vi "svx_Autoscale Ranges.vi"(7 "Plot Area:Size:Width":u32, 10 "Display State In":T4={"X Scale Width %"=50.0, "Y Scale Height %"=50.0, "X-Axis Range"={"Minimum"=0.0, "Maximum"=10.0}, "Y-Axis Range"={"Minimum"=0.0, "Maximum"=10.0}, "Z-Axis Range"={"Minimum"=0.0, "Maximum"=10.0}, "Plot Color"=61212, "Frame Color"=16252785, "Background Color"=16777222, "Initial AutoScale Y"=TRUE, "AutoScale X"=2, "AutoScale Y"=2, "AutoScale Z"=2, "Plot Transparency"=FALSE, "X-Axis Name"="Frequency", "Y-Axis Name"="Amplitude", "Z-Axis Name"="", "X-Axis Scaling Factor"={"Offset"=0.0, "Multiplier"=1.0}, "Y-Axis Scaling Factor"={"Offset"=0.0, "Multiplier"=1.0}, "Z-Axis Scaling Factor"={"Offset"=0.0, "Multiplier"=1.0}, "X-Scale Visible"=TRUE, "Y-Scale Visible"=TRUE, "Z-Scale Visible"=TRUE, "X-Scale Label Visible"=TRUE, "Y-Scale Label Visible"=TRUE, "Z-Scale Label Visible"=TRUE, "X-Axis Range Scaled"={"Minimum"=0.0, "Maximum"=10.0}, "Y-Axis Range Scaled"={"Minimum"=0.0, "Maximum"=10.0}, "Z-Axis Range Scaled"={"Minimum"=0.0, "Maximum"=10.0}, "Rev Z Order"=FALSE, "X-Scale Format Str"="%#.4g", "Y-Scale Format Str"="%#.4g", "Z-Scale Format Str"="%#.4g", "Decor color"=12369084, "Scale Range Change"=refnum, "out of state queue"=refnum, "property nodes"=refnum, "Lines"=[], "Line Properties"={"Line Color"=61212, "Line Width"=61212, "Line Style"=enum."Dash", "DisplayLines"=FALSE}} {"Line Properties"."Line Width" min=1}, 11 "Data Array In":T2={"z0"=0.0, "dz"=1.0, "Plots"=[]}) -> (0 "Cropped Info out":cluster{"First Index":i32, "Length":i32}, 1 "Update Ranges":bool[](array[boolean]), 2 "Display State Out":T4={"X Scale Width %"=50.0, "Y Scale Height %"=50.0, "X-Axis Range"={"Minimum"=0.0, "Maximum"=10.0}, "Y-Axis Range"={"Minimum"=0.0, "Maximum"=10.0}, "Z-Axis Range"={"Minimum"=0.0, "Maximum"=10.0}, "Plot Color"=61212, "Frame Color"=16252785, "Background Color"=16777222, "Initial AutoScale Y"=TRUE, "AutoScale X"=2, "AutoScale Y"=2, "AutoScale Z"=2, "Plot Transparency"=FALSE, "X-Axis Name"="Frequency", "Y-Axis Name"="Amplitude", "Z-Axis Name"="", "X-Axis Scaling Factor"={"Offset"=0.0, "Multiplier"=1.0}, "Y-Axis Scaling Factor"={"Offset"=0.0, "Multiplier"=1.0}, "Z-Axis Scaling Factor"={"Offset"=0.0, "Multiplier"=1.0}, "X-Scale Visible"=TRUE, "Y-Scale Visible"=TRUE, "Z-Scale Visible"=TRUE, "X-Scale Label Visible"=TRUE, "Y-Scale Label Visible"=TRUE, "Z-Scale Label Visible"=TRUE, "X-Axis Range Scaled"={"Minimum"=0.0, "Maximum"=10.0}, "Y-Axis Range Scaled"={"Minimum"=0.0, "Maximum"=10.0}, "Z-Axis Range Scaled"={"Minimum"=0.0, "Maximum"=10.0}, "Rev Z Order"=FALSE, "X-Scale Format Str"="%#.4g", "Y-Scale Format Str"="%#.4g", "Z-Scale Format Str"="%#.4g", "Decor color"=12369084, "Scale Range Change"=refnum, "out of state queue"=refnum, "property nodes"=refnum, "Lines"=[], "Line Properties"={"Line Color"=61212, "Line Width"=61212, "Line Style"=enum."Dash", "DisplayLines"=FALSE}} {"Line Properties"."Line Width" min=1}, 3 "Dec/Cropped and Lines Out":T1={"Dec/Cropped in"={"z0"=0.0, "dz"=1.0, "Plots"=[]}, "Lines"=[]}, 4 "Update Autoscale":bool)   [LabVIEW 2017, in "SVX Waterfall Graph.xctl"]
uses:
  <vilib>/addons/_XControls/Waterfall Graph/SVX Waterfall Graph.xctl
  <vilib>/addons/_XControls/Waterfall Graph/subVIs/svx_Waterfall Data.ctl
  <vilib>/addons/_XControls/Waterfall Graph/subVIs/svx_CroppedData.ctl
  <vilib>/addons/_NISVFA/_Shared subVIs/Controls/svc_Cluster of Array of Cluster of XYZ.ctl
  <vilib>/addons/_XControls/Waterfall Graph/subVIs/svx_Waterfall State.ctl
panel:
  in  "Dec/Cropped and Lines In":T1={"Dec/Cropped in"={"z0"=0.0, "dz"=1.0, "Plots"=[]}, "Lines"=[]}
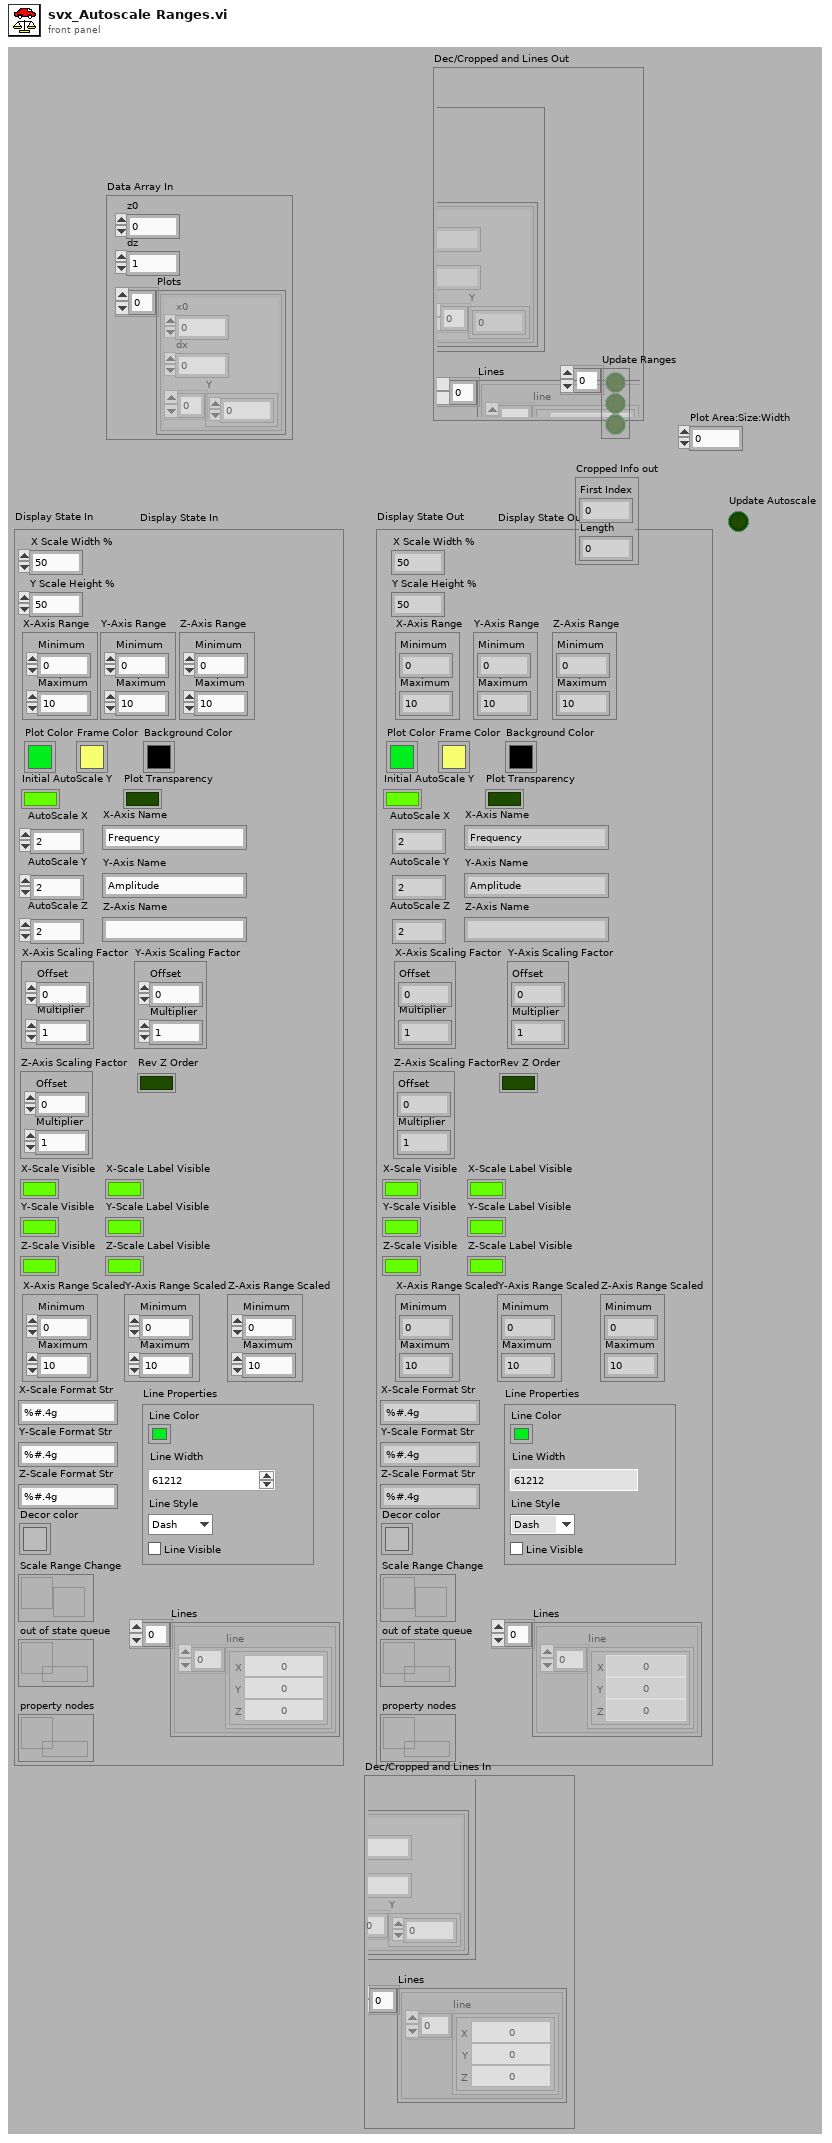
[diagram p1: front panel]
types:
  T1 = typedef "SVX Waterfall Graph.xctl/svx_CroppedData.ctl" = cluster{"Dec/Cropped in":T2, "Lines":T3[]}
  T2 = typedef "SVX Waterfall Graph.xctl/svx_Waterfall Data.ctl" = cluster{"z0":dbl, "dz":dbl, "Plots":cluster{"x0":dbl, "dx":dbl, "Y":dbl[]}[]}
  T3 = typedef "svc_Cluster of Array of Cluster of XYZ.ctl" = cluster{"line":cluster{"X":dbl, "Y":dbl, "Z":dbl}[]}
  T4 = typedef "SVX Waterfall Graph.xctl/svx_Waterfall State.ctl" = cluster{"X Scale Width %":dbl, "Y Scale Height %":dbl, "X-Axis Range":cluster{"Minimum":dbl, "Maximum":dbl}, "Y-Axis Range":cluster{"Minimum":dbl, "Maximum":dbl}, "Z-Axis Range":cluster{"Minimum":dbl, "Maximum":dbl}, "Plot Color":u32, "Frame Color":u32, "Background Color":u32, "Initial AutoScale Y":bool, "AutoScale X":u8, "AutoScale Y":u8, "AutoScale Z":u8, "Plot Transparency":bool, "X-Axis Name":string, "Y-Axis Name":string, "Z-Axis Name":string, "X-Axis Scaling Factor":cluster{"Offset":dbl, "Multiplier":dbl}, "Y-Axis Scaling Factor":cluster{"Offset":dbl, "Multiplier":dbl}, "Z-Axis Scaling Factor":cluster{"Offset":dbl, "Multiplier":dbl}, "X-Scale Visible":bool, "Y-Scale Visible":bool, "Z-Scale Visible":bool, "X-Scale Label Visible":bool, "Y-Scale Label Visible":bool, "Z-Scale Label Visible":bool, "X-Axis Range Scaled":cluster{"Minimum":dbl, "Maximum":dbl}, "Y-Axis Range Scaled":cluster{"Minimum":dbl, "Maximum":dbl}, "Z-Axis Range Scaled":cluster{"Minimum":dbl, "Maximum":dbl}, "Rev Z Order":bool, "X-Scale Format Str":string, "Y-Scale Format Str":string, "Z-Scale Format Str":string, "Decor color":u32, "Scale Range Change":refnum<user-event>, "out of state queue":refnum<queue>, "property nodes":refnum<queue>, "Lines":T3[], "Line Properties":cluster{"Line Color":u32, "Line Width":u16, "Line Style":enum32{"Solid", "Dash", "Dot", "DashDot", "DashDotDot"}, "DisplayLines":bool}}
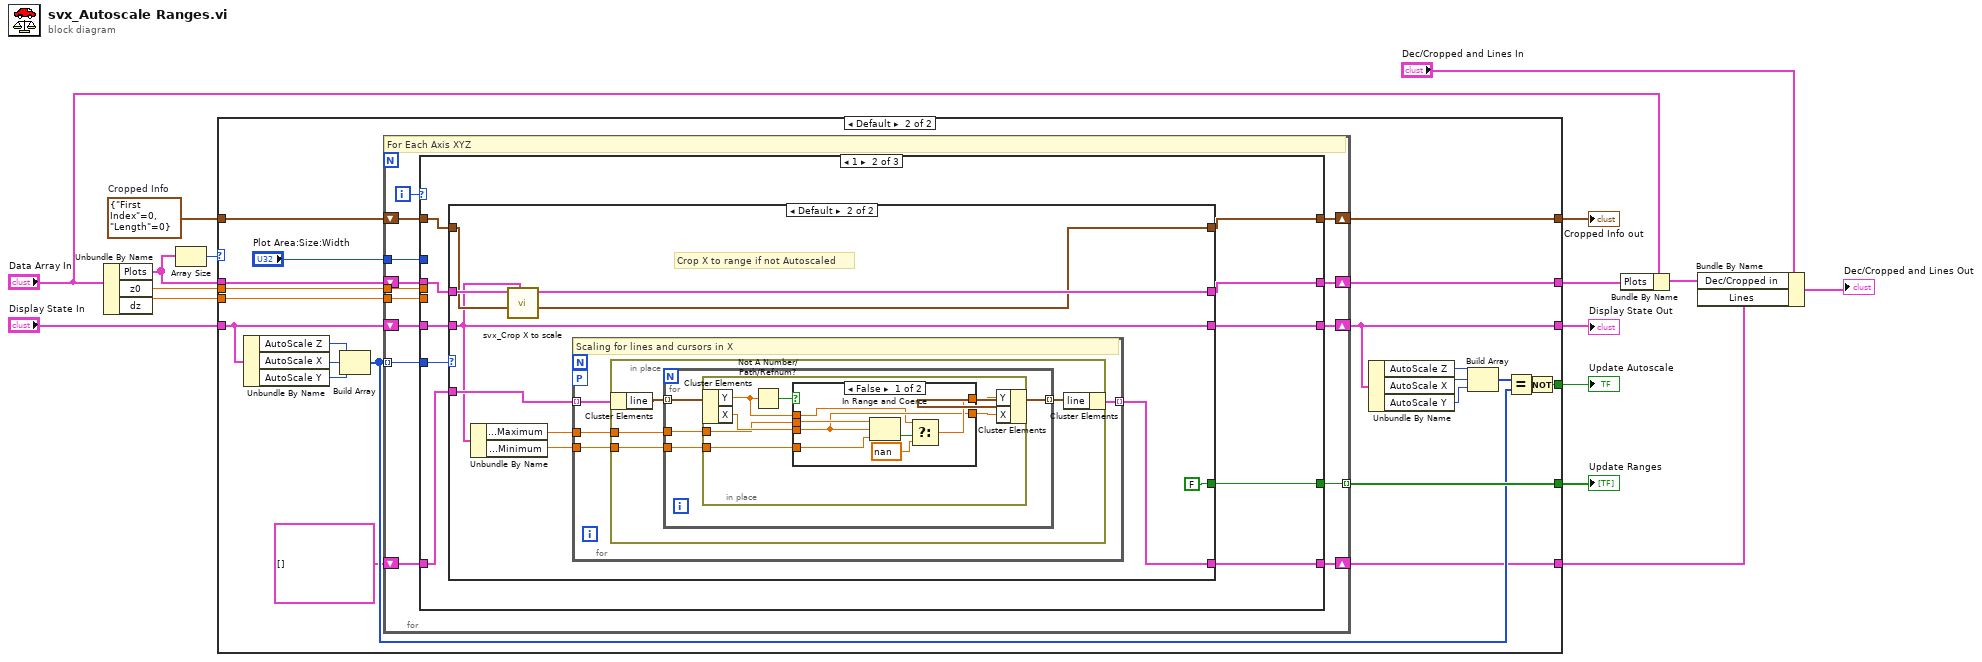
[diagram p0: block diagram]
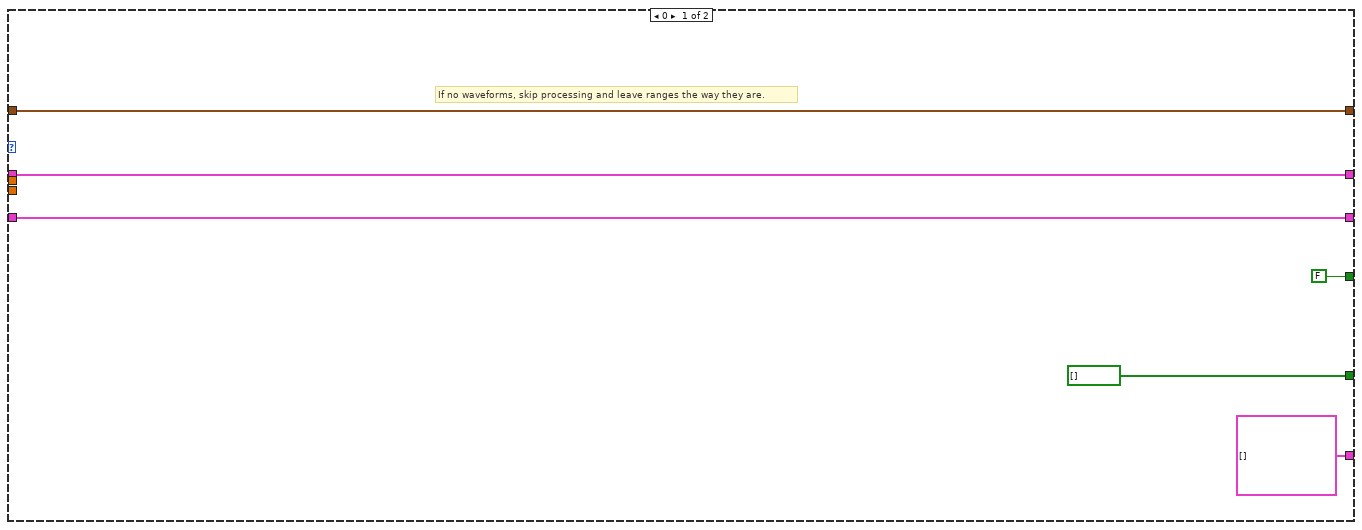
[diagram p2: hidden frame]
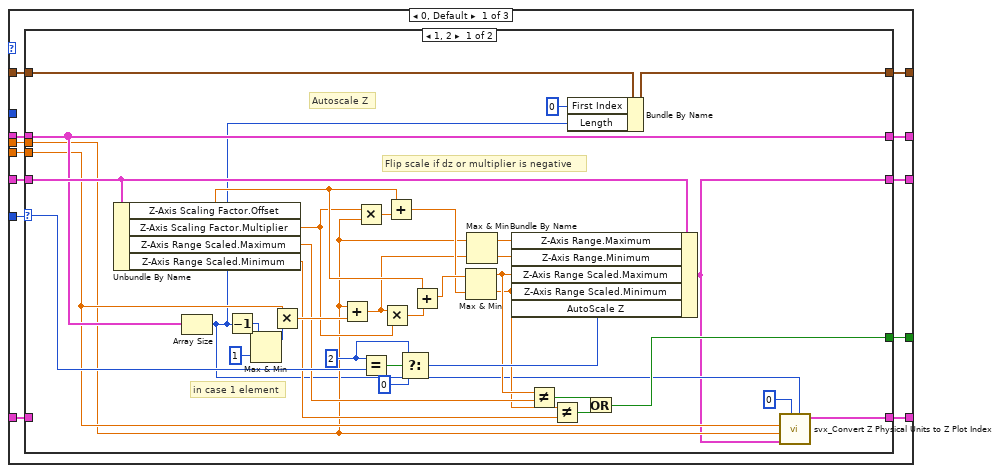
[diagram p3: hidden frame]
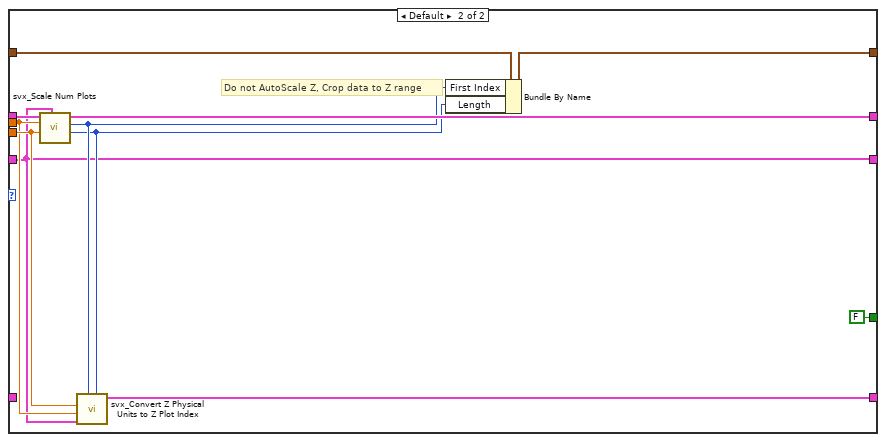
[diagram p4: hidden frame]
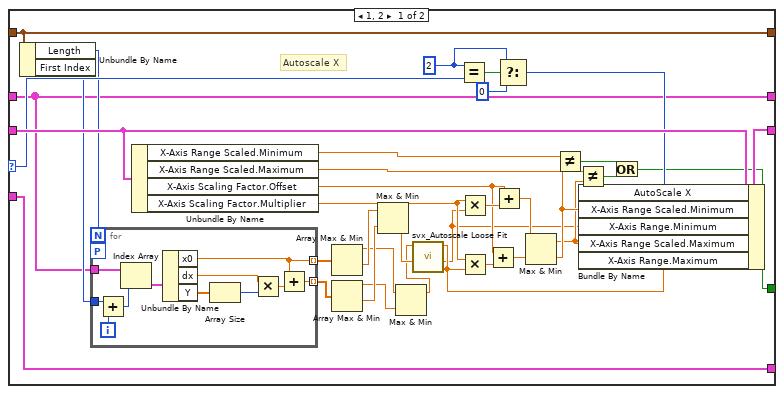
[diagram p5: hidden frame]
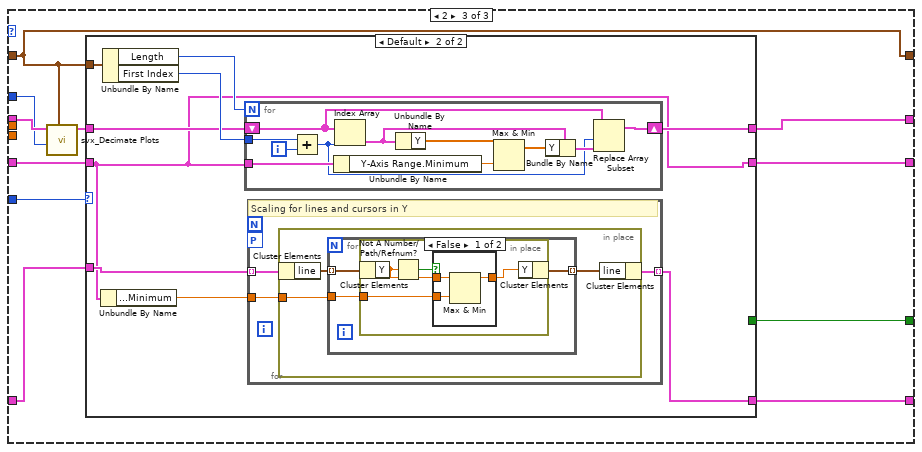
[diagram p7: hidden frame]
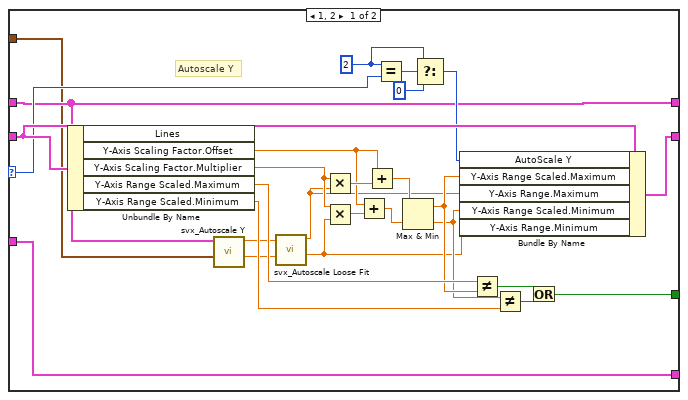
[diagram p8: hidden frame]
diagram:
  w12 = cluster{"First Index":i32, "Length":i32} {"First Index"=0, "Length"=0}  # Cropped Info
  n1 = Unbundle By Name("Data Array In") -> ("Plots"=w11:cluster{"x0":dbl, "dx":dbl, "Y":dbl[]}[], "z0"=w8:dbl, "dz"=w7:dbl)
  n2 = Array Size(array=w11) -> (size(s)=w15:i32)
  n3 = case shown="Default" w15 {
    tunnel: [w21 w30] -> w2
    tunnel: "Display State In" -> [w21 w44]
    tunnel: w11 -> [w22 w40]
    tunnel: [w22 w39] -> w9
    tunnel: [bool[] [] w38] -> w14
    tunnel: [w19 w37] -> w13
    tunnel: w12 -> [w19 w36]
    tunnel: w8 -> [_ w25]
    tunnel: w7 -> [_ w26]
    tunnel: [FALSE w27] -> w6
    tunnel: [T3[] [] ("Lines") w23] -> w1
    frame 0 {
      # "If no waveforms, skip processing and leave ranges the way they are."
    }
    frame Default {
      n4 = Unbundle By Name(w44) -> ("AutoScale Z"=w43:u8, "AutoScale X"=w42:u8, "AutoScale Y"=w41:u8)
      n5 = Build Array(w43, w42, w41) -> (w29:u8[])
      n6 = for {
        shift-right: [w47] -> w30
        shift-left: w44 -> [w58]
        tunnel: w29 -> [w55] mode=indexing
        shift-right: [w54] -> w39
        shift-left: w40 -> [w57]
        tunnel: [w53] -> w38 mode=indexing
        shift-right: [w51] -> w37
        shift-left: w36 -> [w52]
        tunnel: w25 -> [w50]
        tunnel: w26 -> [w48]
        tunnel: "Plot Area:Size:Width" -> [w49]
        shift-right: [w46] -> w23
        shift-left: T3[] [] ("Lines") -> [w45]
        i -> [w56]
        # "For Each Axis XYZ"
        n7 = case shown="1" w56 {
          tunnel: w58 -> [w70 w127 w222]
          tunnel: [w69 w120 w221] -> w47
          tunnel: w57 -> [w68 w126 w217]
          tunnel: w55 -> [w67 w125 w220]
          tunnel: [w66 w124 w219] -> w54
          tunnel: [w65 w123 w218] -> w53
          tunnel: w52 -> [w64 w122 w215]
          tunnel: [w63 w121 w215] -> w51
          tunnel: w50 -> [w62 _ _]
          tunnel: w48 -> [w61 _ _]
          tunnel: w49 -> [_ _ w214]
          tunnel: [w60 w118 w212] -> w46
          tunnel: w45 -> [w59 w119 w213]
          frame 0, Default {
            n8 = case shown="1, 2" w67 {
              selector: w67 -> [w92 _]
              tunnel: w70 -> [w106 w107]
              tunnel: [w71 w107] -> w69
              tunnel: w68 -> [w80 w117]
              tunnel: [w80 w116] -> w66
              tunnel: [w84 FALSE] -> w65
              tunnel: w64 -> [w83 w114]
              tunnel: [w82 w113] -> w63
              tunnel: w62 -> [w75 w111]
              tunnel: w61 -> [w76 w112]
              tunnel: [w72 w108] -> w60
              tunnel: w59 -> [_ _]
              frame 1, 2 {
                w94 = u8 2 ("AutoScale Y")
                # "in case 1 element"
                # "Flip scale if dz or multiplier is negative"
                # "Autoscale Z"
                n9 = Unbundle By Name(w106) -> ("Z-Axis Scaling Factor.Offset"=w103:dbl, "Z-Axis Scaling Factor.Multiplier"=w101:dbl, "Z-Axis Range Scaled.Maximum"=w88:dbl, "Z-Axis Range Scaled.Minimum"=w86:dbl)
                n10 = Array Size(array=w80) -> (size(s)=w73:i32)
                n11 = Decrement(x=w73) -> (x-1=w79:i32)
                n12 = Max & Min(x=w79, y=1) -> (max(x,y)=w78:i32)  [unwired: 1 out]
                n13 = Multiply(x=w76, y=w78) -> (x*y=w102:dbl)
                n14 = Add(x=w75, y=w102) -> (x+y=w98:dbl)
                n15 = Multiply(x=w101, y=w75) -> (x*y=w105:dbl)
                n16 = Equal?(x=w94, y=w92) -> (x = y?=w95:bool)
                n17 = Multiply(x=w98, y=w101) -> (x*y=w104:dbl)
                n18 = Add(x=w103, y=w105) -> (x+y=w99:dbl)
                n19 = Select(t=w94, s=w95, f=u8 0 ("AutoScale Y")) -> (s? t:f=w91:u8)
                n20 = Add(x=w103, y=w104) -> (x+y=w100:dbl)
                n21 = Max & Min(x=w100, y=w99) -> (max(x,y)=w87:dbl, min(x,y)=w85:dbl)
                n22 = Max & Min(x=w75, y=w98) -> (max(x,y)=w97:dbl, min(x,y)=w96:dbl)
                n23 = Bundle By Name(cluster=w106, "Z-Axis Range.Maximum"=w97, "Z-Axis Range.Minimum"=w96, "Z-Axis Range Scaled.Maximum"=w87, "Z-Axis Range Scaled.Minimum"=w85, "AutoScale Z"=w91) -> (w71:T4)
                n24 = Not Equal?(x=w87, y=w88) -> (x != y?=w90:bool)
                n25 = Not Equal?(x=w85, y=w86) -> (x != y?=w89:bool)
                n26 = Bundle By Name(cluster=w83, "First Index"=0, "Length"=w73) -> (w82:cluster{"First Index":i32, "Length":i32})
                n27 = Or(x=w90, y=w89) -> (x .or. y?=w84:bool)
                n28 = call <vilib>:"svx_Convert Z Physical Units to Z Plot Index.vi"("Z length"=w73, "Z Index"=0 ("First Index"), "Display State In"=w71, "z0"=w75, "dz"=w76) -> ("Lines"=w72:T3[])  [unwired: 6 in]
              }
              frame Default {
                # "Do not AutoScale Z, Crop data to Z range"
                n29 = call <vilib>:"svx_Scale Num Plots.vi"("Display State In"=w107, "dz"=w112, "z0"=w111, "Plots"=w117) -> ("Z length"=w109:i32, "Z Index"=w110:i32, "Plots out"=w116:cluster{"x0":dbl, "dx":dbl, "Y":dbl[]}[])  [unwired: 5 in]
                n30 = call <vilib>:"svx_Convert Z Physical Units to Z Plot Index.vi"("Z length"=w109, "Z Index"=w110, "Display State In"=w107, "z0"=w111, "dz"=w112) -> ("Lines"=w108:T3[])  [unwired: 6 in]
                n31 = Bundle By Name(cluster=w114, "First Index"=w110, "Length"=w109) -> (w113:cluster{"First Index":i32, "Length":i32})
              }
            }
          }
          frame 1 {
            n32 = case shown="Default" w125 {
              selector: w125 -> [w145 _]
              tunnel: w127 -> [w161 w174]
              tunnel: [w162 w174] -> w120
              tunnel: w126 -> [w129 w180]
              tunnel: [w129 w183] -> w124
              tunnel: [w138 FALSE ("Boolean")] -> w123
              tunnel: w122 -> [w136 w177]
              tunnel: [w136 w181] -> w121
              tunnel: w119 -> [w128 w176]
              tunnel: [w128 w175] -> w118
              frame 1, 2 {
                w147 = u8 2 ("AutoScale Y")
                # "Autoscale X"
                n33 = Unbundle By Name(w136) -> ("Length"=w135:i32, "First Index"=w134:i32)
                n34 = for {
                  N: w135 -> [_]
                  tunnel: [w169] -> w154 mode=indexing
                  tunnel: [w168] -> w153 mode=indexing
                  tunnel: w129 -> [w167]
                  tunnel: w134 -> [w164]
                  workers-P: _ -> [_]
                  i -> [w165]
                  n35 = Add(x=w164, y=w165) -> (x+y=w163:i32)
                  n36 = Index Array(array=w167, index=w163) -> (element=w166:cluster{"x0":dbl, "dx":dbl, "Y":dbl[]})
                  n37 = Unbundle By Name(w166) -> ("x0"=w169:dbl, "dx"=w171:dbl, "Y"=w173:dbl[])
                  n38 = Array Size(array=w173) -> (size(s)=w172:i32)
                  n39 = Multiply(x=w171, y=w172) -> (x*y=w170:dbl)
                  n40 = Add(x=w169, y=w170) -> (x+y=w168:dbl)
                }
                n41 = Unbundle By Name(w161) -> ("X-Axis Range Scaled.Minimum"=w137:dbl, "X-Axis Range Scaled.Maximum"=w142:dbl, "X-Axis Scaling Factor.Offset"=w157:dbl, "X-Axis Scaling Factor.Multiplier"=w158:dbl)
                n42 = Array Max & Min(array=w154) -> (max value=w150:dbl, min value=w152:dbl)  [unwired: 2 out]
                n43 = Array Max & Min(array=w153) -> (max value=w149:dbl, min value=w151:dbl)  [unwired: 2 out]
                n44 = Max & Min(x=w152, y=w151) -> (min(x,y)=w133:dbl)  [unwired: 1 out]
                n45 = Max & Min(x=w150, y=w149) -> (max(x,y)=w132:dbl)  [unwired: 1 out]
                n46 = call <vilib>:"svx_Autoscale Loose Fit.vi"("Min"=w133, "Max"=w132) -> ("Loose Fit Min"=w130:dbl, "Loose Fit Max"=w131:dbl)  [unwired: 8 in]
                n47 = Equal?(x=w147, y=w145) -> (x = y?=w148:bool)
                n48 = Multiply(x=w158, y=w130) -> (x*y=w160:dbl)
                n49 = Multiply(x=w158, y=w131) -> (x*y=w159:dbl)
                n50 = Add(x=w157, y=w159) -> (x+y=w156:dbl)
                n51 = Add(x=w157, y=w160) -> (x+y=w155:dbl)
                n52 = Select(t=w147, s=w148, f=u8 0 ("AutoScale Y")) -> (s? t:f=w144:u8)
                n53 = Max & Min(x=w155, y=w156) -> (max(x,y)=w141:dbl, min(x,y)=w143:dbl)
                n54 = Not Equal?(x=w137, y=w143) -> (x != y?=w140:bool)
                n55 = Not Equal?(x=w142, y=w141) -> (x != y?=w139:bool)
                n56 = Bundle By Name(cluster=w161, "AutoScale X"=w144, "X-Axis Range Scaled.Minimum"=w143, "X-Axis Range.Minimum"=w130, "X-Axis Range Scaled.Maximum"=w141, "X-Axis Range.Maximum"=w131) -> (w162:T4)
                n57 = Or(x=w140, y=w139) -> (x .or. y?=w138:bool)
              }
              frame Default {
                # "Crop X to range if not Autoscaled"
                n58 = Unbundle By Name(w174) -> ("X-Axis Range.Maximum"=w179:dbl, "X-Axis Range.Minimum"=w178:dbl)
                n59 = call <vilib>:"svx_Crop X to scale.vi"("Display State In"=w174, "Cropped Info"=w177, "Plots"=w180) -> ("Cropped Info out"=w181:cluster{"First Index":i32, "Length":i32}, "Plots"=w183:cluster{"x0":dbl, "dx":dbl, "Y":dbl[]}[])  [unwired: 7 in]
                n60 = for {
                  tunnel: w176 -> [w186] mode=indexing
                  tunnel: w179 -> [w187]
                  tunnel: [w185] -> w175 mode=indexing
                  tunnel: w178 -> [w184]
                  workers-P: _ -> [_]
                  # "Scaling for lines and cursors in X"
                  n61 = in-place {
                    in-place-border: w187 -> [w191]
                    in-place-border: w184 -> [w188]
                    n62 = in-place-cluster #1(w186) -> ("line"=w190:cluster{"X":dbl, "Y":dbl, "Z":dbl}[])
                    n63 = for {
                      tunnel: w190 -> [w195] mode=indexing
                      tunnel: w191 -> [w194]
                      tunnel: [w193] -> w189 mode=indexing
                      tunnel: w188 -> [w192]
                      n64 = in-place {
                        in-place-border: w194 -> [w198]
                        in-place-border: w192 -> [w197]
                        n65 = in-place-cluster #2(w195) -> ("Y"=w201:dbl, "X"=w199:dbl)
                        n66 = Not A Number/Path/Refnum?(number/path/refnum=w201) -> (NaN/Path/Refnum?=w202:bool)
                        n67 = case shown="False" w202 {
                          tunnel: w201 -> [w203 w211]
                          tunnel: [w208 w211] -> w200
                          tunnel: w199 -> [w204 w210]
                          tunnel: w198 -> [w206 _]
                          tunnel: w197 -> [w207 _]
                          tunnel: [w204 w210] -> w196
                          frame False {
                            n68 = In Range and Coerce(upper limit=w206, x=w204, lower limit=w207) -> (In Range?=w209:bool)  [unwired: 1 out]
                            n69 = Select(t=w203, s=w209, f=nan) -> (s? t:f=w208:dbl)
                          }
                          frame True {
                            # "Y is NaN"
                          }
                        }
                        n70 = in-place-cluster #2("Y"=w200, "X"=w196) -> (w193:cluster{"X":dbl, "Y":dbl, "Z":dbl})
                      }
                    }
                    n71 = in-place-cluster #1("line"=w189) -> (w185:T3)
                  }
                }
              }
            }
          }
          frame 2 {
            n72 = call <vilib>:"svx_Decimate Plots.vi"("Cropped Info"=w215, "Width"=w214, "Plots"=w217) -> ("Plots out"=w216:cluster{"x0":dbl, "dx":dbl, "Y":dbl[]}[])  [unwired: 8 in]
            n73 = case shown="Default" w220 {
              selector: w220 -> [w241 _]
              tunnel: w222 -> [w248 w251]
              tunnel: [w249 w251] -> w221
              tunnel: w216 -> [w227 w254]
              tunnel: [w227 w255] -> w219
              tunnel: [w230 FALSE] -> w218
              tunnel: w215 -> [w226 w258]
              tunnel: w213 -> [w223 w252]
              tunnel: [w223 w250] -> w212
              frame 1, 2 {
                w239 = u8 2 ("AutoScale Y")
                # "Autoscale Y"
                n74 = Unbundle By Name(w248) -> ("Y-Axis Scaling Factor.Offset"=w244:dbl, "Y-Axis Scaling Factor.Multiplier"=w245:dbl, "Y-Axis Range Scaled.Maximum"=w234:dbl, "Y-Axis Range Scaled.Minimum"=w232:dbl)  [unwired: 1 out]
                n75 = call <vilib>:"svx_Autoscale Y.vi"("Cropped Info"=w226, "Plots"=w227) -> ("min"=w224:dbl, "max"=w225:dbl)  [unwired: 8 in]
                n76 = call <vilib>:"svx_Autoscale Loose Fit.vi"("Min"=w224, "Max"=w225) -> ("Loose Fit Min"=w228:dbl, "Loose Fit Max"=w229:dbl)  [unwired: 8 in]
                n77 = Multiply(x=w245, y=w229) -> (x*y=w247:dbl)
                n78 = Multiply(x=w245, y=w228) -> (x*y=w246:dbl)
                n79 = Add(x=w244, y=w246) -> (x+y=w243:dbl)
                n80 = Add(x=w244, y=w247) -> (x+y=w242:dbl)
                n81 = Equal?(x=w239, y=w241) -> (x = y?=w240:bool)
                n82 = Max & Min(x=w242, y=w243) -> (max(x,y)=w233:dbl, min(x,y)=w231:dbl)
                n83 = Select(t=w239, s=w240, f=u8 0 ("AutoScale Y")) -> (s? t:f=w237:u8)
                n84 = Bundle By Name(cluster=w248, "AutoScale Y"=w237, "Y-Axis Range Scaled.Maximum"=w233, "Y-Axis Range.Maximum"=w229, "Y-Axis Range Scaled.Minimum"=w231, "Y-Axis Range.Minimum"=w228) -> (w249:T4)
                n85 = Not Equal?(x=w234, y=w233) -> (x != y?=w236:bool)
                n86 = Not Equal?(x=w231, y=w232) -> (x != y?=w235:bool)
                n87 = Or(x=w236, y=w235) -> (x .or. y?=w230:bool)
              }
              frame Default {
                n88 = Unbundle By Name(w251) -> ("Y-Axis Range.Minimum"=w253:dbl)
                n89 = Unbundle By Name(w258) -> ("Length"=w257:i32, "First Index"=w256:i32)
                n90 = for {
                  N: w257 -> [_]
                  tunnel: w251 -> [w287]
                  tunnel: w256 -> [w281]
                  shift-right: [w279] -> w255
                  shift-left: w254 -> [w278]
                  i -> [w282]
                  n91 = Add(x=w281, y=w282) -> (x+y=w277:i32)
                  n92 = Unbundle By Name(w287) -> ("Y-Axis Range.Minimum"=w285:dbl)
                  n93 = Index Array(array=w278, index=w277) -> (element=w283:cluster{"x0":dbl, "dx":dbl, "Y":dbl[]})
                  n94 = Unbundle By Name(w283) -> ("Y"=w286:dbl[])
                  n95 = Max & Min(x=w286, y=w285) -> (max(x,y)=w284:dbl[])  [unwired: 1 out]
                  n96 = Bundle By Name(cluster=w283, "Y"=w284) -> (w280:cluster{"x0":dbl, "dx":dbl, "Y":dbl[]})
                  n97 = Replace Array Subset(array=w278, new element=w280, index=w277) -> (w279:cluster{"x0":dbl, "dx":dbl, "Y":dbl[]}[])
                }
                n98 = for {
                  tunnel: w252 -> [w261] mode=indexing
                  tunnel: w253 -> [w262]
                  tunnel: [w260] -> w250 mode=indexing
                  workers-P: _ -> [_]
                  # "Scaling for lines and cursors in Y"
                  n99 = in-place {
                    in-place-border: w262 -> [w265]
                    n100 = in-place-cluster #3(w261) -> ("line"=w264:cluster{"X":dbl, "Y":dbl, "Z":dbl}[])
                    n101 = for {
                      tunnel: w264 -> [w268] mode=indexing
                      tunnel: w265 -> [w267]
                      tunnel: [w266] -> w263 mode=indexing
                      n102 = in-place {
                        in-place-border: w267 -> [w269]
                        n103 = in-place-cluster #4(w268) -> ("Y"=w271:dbl)
                        n104 = Not A Number/Path/Refnum?(number/path/refnum=w271) -> (NaN/Path/Refnum?=w272:bool)
                        n105 = case shown="False" w272 {
                          tunnel: w271 -> [w275 w276]
                          tunnel: [w273 w276] -> w270
                          tunnel: w269 -> [w274 _]
                          frame False {
                            n106 = Max & Min(x=w275, y=w274) -> (max(x,y)=w273:dbl)  [unwired: 1 out]
                          }
                          frame True {
                            # "NaN"
                          }
                        }
                        n107 = in-place-cluster #4("Y"=w270) -> (w266:cluster{"X":dbl, "Y":dbl, "Z":dbl})
                      }
                    }
                    n108 = in-place-cluster #3("line"=w263) -> (w260:T3)
                  }
                }
              }
            }
          }
        }
      }
      n109 = Unbundle By Name(w30) -> ("AutoScale Z"=w33:u8, "AutoScale X"=w32:u8, "AutoScale Y"=w31:u8)
      n110 = Build Array(w33, w32, w31) -> (w34:u8[])
      n111 = Equal?(x=w34, y=w29) -> (x = y?=w28:bool)
      n112 = Not(x=w28) -> (.not. x?=w27:bool)
    }
  }
  "Display State Out" <- w2
  "Update Ranges" <- w14
  "Cropped Info out" <- w13
  "Update Autoscale" <- w6
  n113 = Bundle By Name(cluster="Data Array In", "Plots"=w9) -> (w4:T2)
  n114 = Bundle By Name(cluster="Dec/Cropped and Lines In", "Dec/Cropped in"=w4, "Lines"=w1) -> (→"Dec/Cropped and Lines Out":T1)
